vi "onStart.vi"(8 "error in (no error)":errorcluster, 11 "DAQ":refnum<class "DAQ.lvclass">) -> (0 "error out":errorcluster, 3 "DAQ out":refnum<class "DAQ.lvclass">)   [LabVIEW 2016, in "DAQ.lvclass"]
doc: "JKI State Machine Objects (SMO) 1.2.1.55\nJKI - JKI\nCopyright (c) 2017, JKI"
uses:
  DAQ.lvclass
  <vilib>/JKI/JKI SMO/SMO/SMO.lvclass
panel:
  # "For instructions on how to use the JKI State Machine Objects, examples and video tutorials, visit:\nhttp://jki.net/state-machine-objects/\n\nJKI State Machine Objects™\nhttp://jki.net/state-machine-objects/\nCopyright (C) 2005-2015, JKI <info@jki.net>\nALL RIGHTS RESERVED"
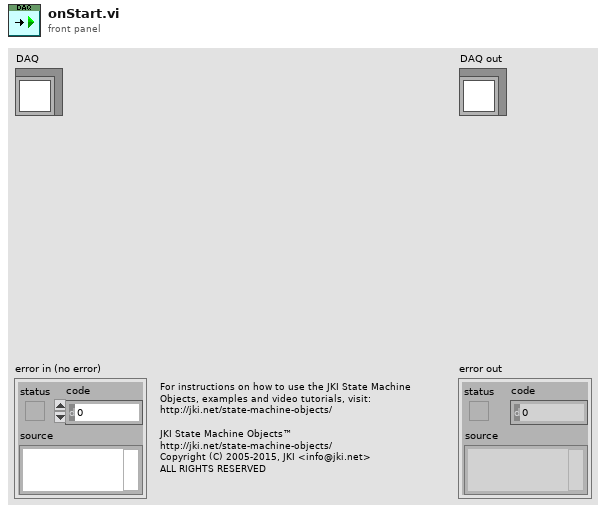
[diagram p1: front panel]
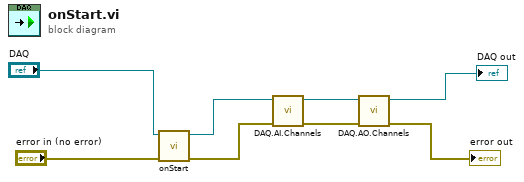
[diagram p0: block diagram]
diagram:
  n1 = call-parent "onStart.vi"("error in (no error)"="error in (no error)", "SMO"="DAQ") -> ("error out"=w6:errorcluster, "SMO out"=w4:refnum<class "DAQ.lvclass">)  [unwired: 8 in]
  n2 = call "DAQ.AI.Channels.vi"("error in (no error)"=w6, "DAQ"=w4) -> ("error out"=w5:errorcluster, "DAQ out"=w3:refnum<class "DAQ.lvclass">)  [unwired: 8 in]
  n3 = call "DAQ.AO.Channels.vi"("error in (no error)"=w5, "DAQ"=w3) -> ("error out"=→"error out":errorcluster, "DAQ out"=→"DAQ out":refnum<class "DAQ.lvclass">)  [unwired: 8 in]
